vi "auto_alignment.vi"(0 "meter-visa":refnum<visa-resource-name>, 1 "xStart":dbl=264.0 format="%#_13g", 2 "yStart":dbl=123.0 format="%#_13g", 3 "NM-params":T1={"alpha"=1.0, "gamma"=2.0, "rho"=0.5, "sigma"=0.5, "simplex L"=0.5}, 5 "PD Values":cluster{"PD1":dbl, "PD2":dbl, "PD3":dbl}, 7 "stage-refs":T2, 9 "meter-error-in":errorcluster, 11 "stage-error-in":errorcluster) -> (4 "Optimized Location":dbl[](array[numeric]), 6 "Pts Tested":dbl[][](array[numeric]), 8 "std dev of simplex values":dbl, 10 "meter-error-out":errorcluster, 14 "run time (min)":dbl, 15 "stage-error-out":errorcluster)   [LabVIEW 2024]
uses:
  O:/DSG/Tyler/EIC/DIRC/daq/automated/Thorlabs.MotionControl.IntegratedStepperMotorsCLI.dll
  Thorlabs.MotionControl.IntegratedStepperMotorsCLI.dll
  O:/DSG/Tyler/EIC/DIRC/daq/automated/Thorlabs.MotionControl.Benchtop.StepperMotorCLI.dll
  Thorlabs.MotionControl.Benchtop.StepperMotorCLI.dll
  5b59031f-b1ff-41af-80a7-e72a33ebffa1.vi
  <vilib>/Array/Sort 2D Array - Pop Stack.vi
  <vilib>/Array/Sort 2D Array - Push Stack.vi
  5b59031f-b1ff-41af-80a7-e72a33ebffa1.vi/269d4b3b-47f5-49e3-8884-44851e4dd9d5.vi
  5b59031f-b1ff-41af-80a7-e72a33ebffa1.vi/6d99389c-673d-4efb-bf33-19b32bcf4cf8.vi
  <vilib>/Analysis/NI_AALBase.lvlib
panel:
  in  "nSamples":dbl=10.0 caption="# Samples"
  in  "simplex-limit":dbl=1e-06 caption="Simplex Length Convergence Goal" format="%#_13g"
  in  "value-limit":dbl=1e-08 caption="Value Convergence Goal" format="%#_13g"
  out "x_c":dbl[](array[numeric])
  out "x_e":dbl[](array[numeric])
  out "x_r":dbl[](array[numeric])
  out "x_o":dbl[](array[numeric])
  out "iterations timeout":bool
  out "simplex converge":bool
  out "value converge":bool
  out "simplex leg lengths":dbl[](array[numeric])
  in  "stop":bool
  # "centroid"
  # "reflection point"
  # "expansion point"
  # "contraction point"
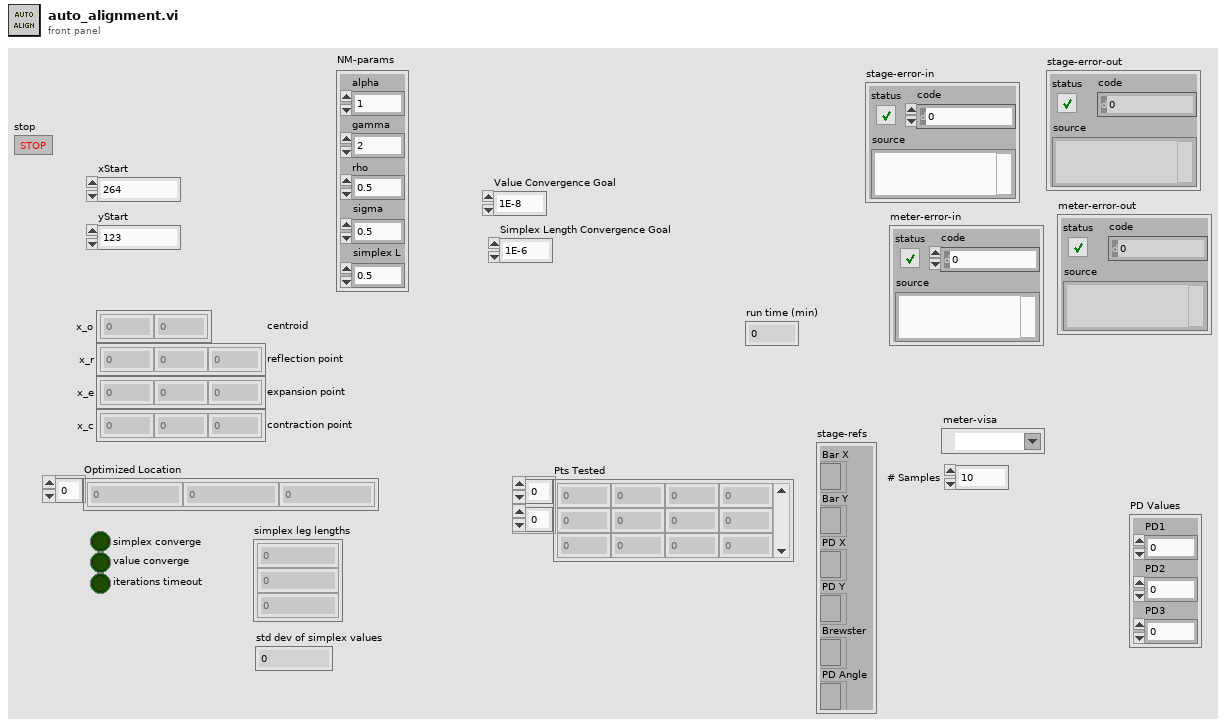
[diagram p1: front panel]
types:
  T1 = cluster{"alpha":dbl, "gamma":dbl, "rho":dbl, "sigma":dbl, "simplex L":dbl}
  T2 = cluster{"Bar X":refnum<k24>, "Bar Y":refnum<k24>, "PD X":refnum<k24>, "PD Y":refnum<k24>, "Brewster":refnum<k24>, "PD Angle":refnum<k24>}
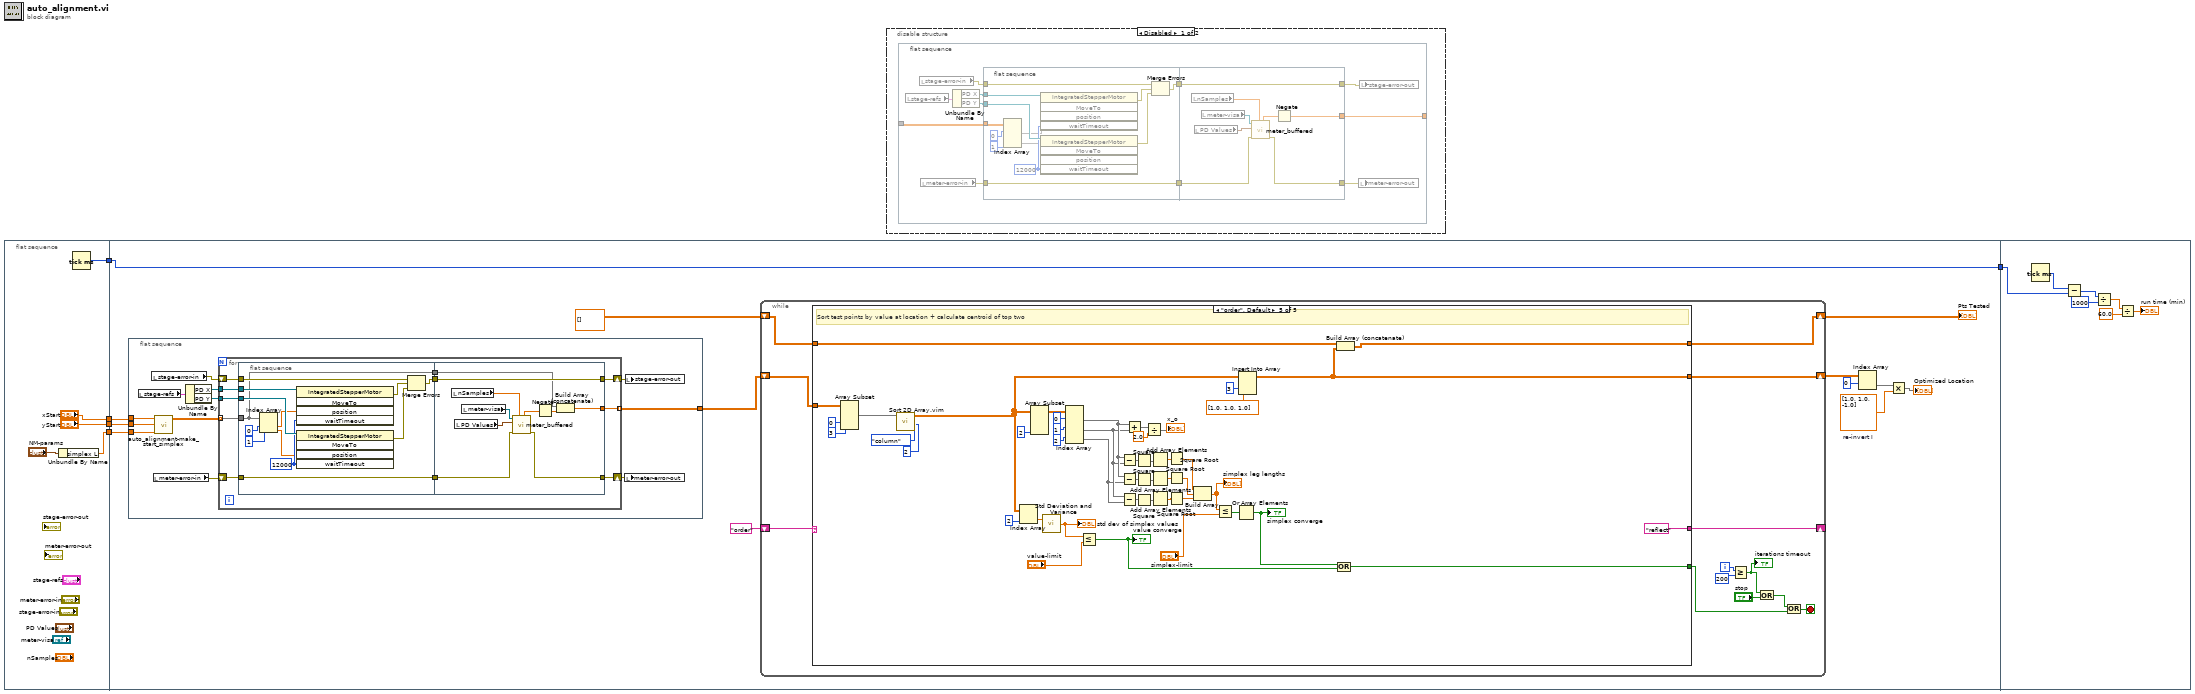
[diagram p0: block diagram]
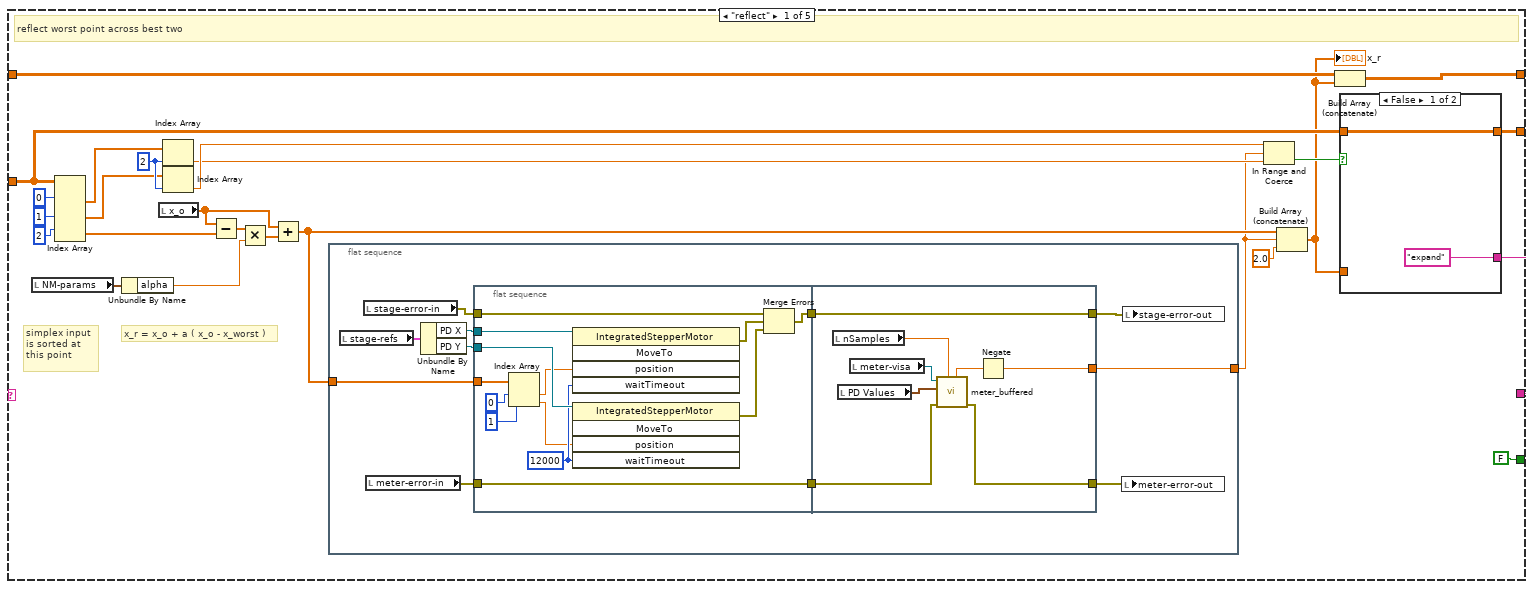
[diagram p3: hidden frame]
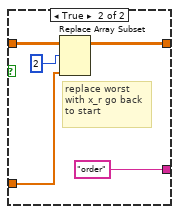
[diagram p4: hidden frame]
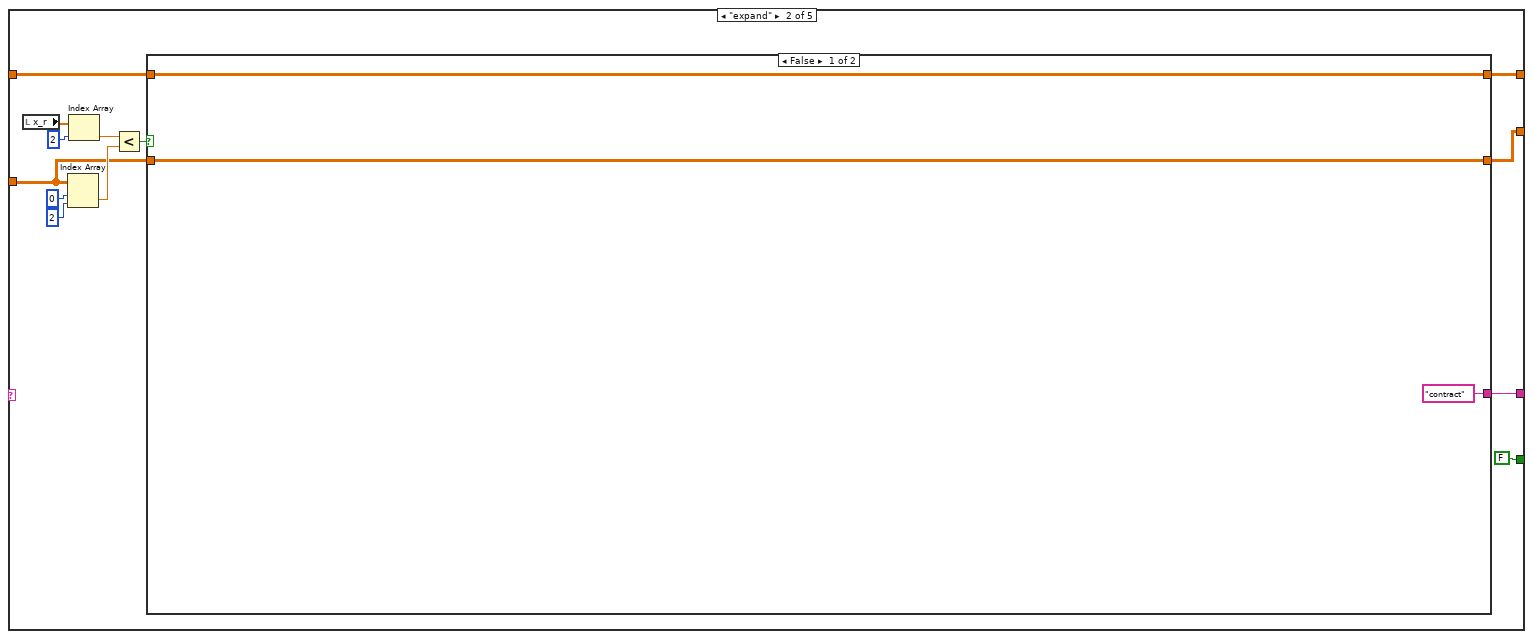
[diagram p5: hidden frame]
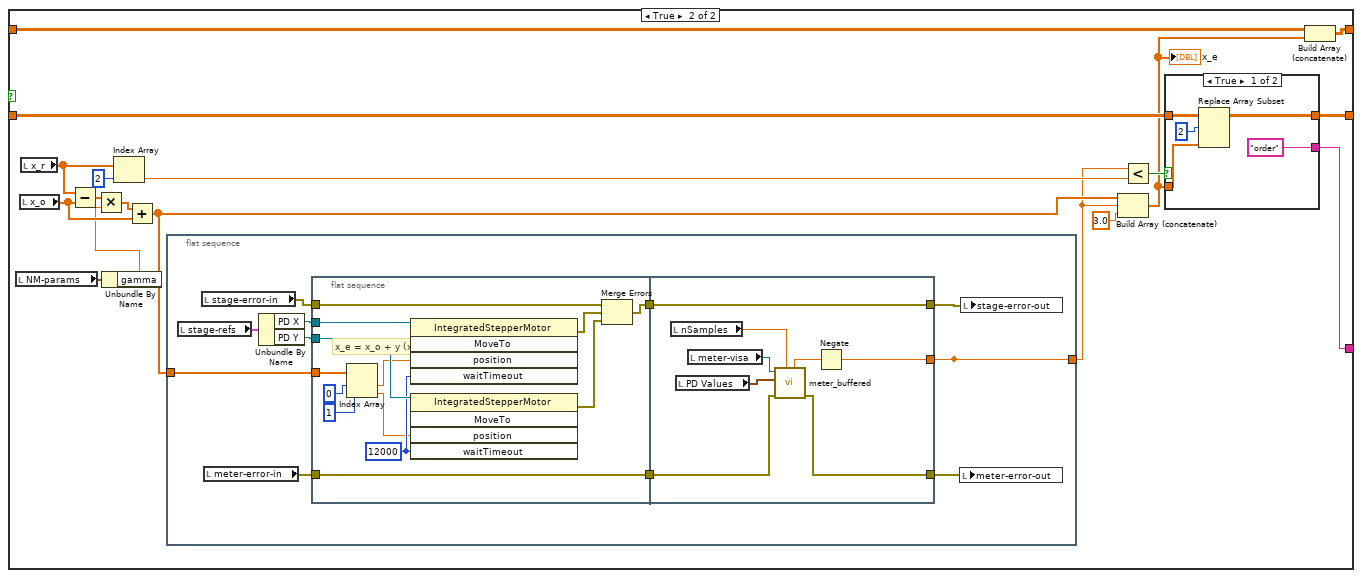
[diagram p6: hidden frame]
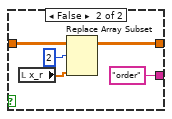
[diagram p7: hidden frame]
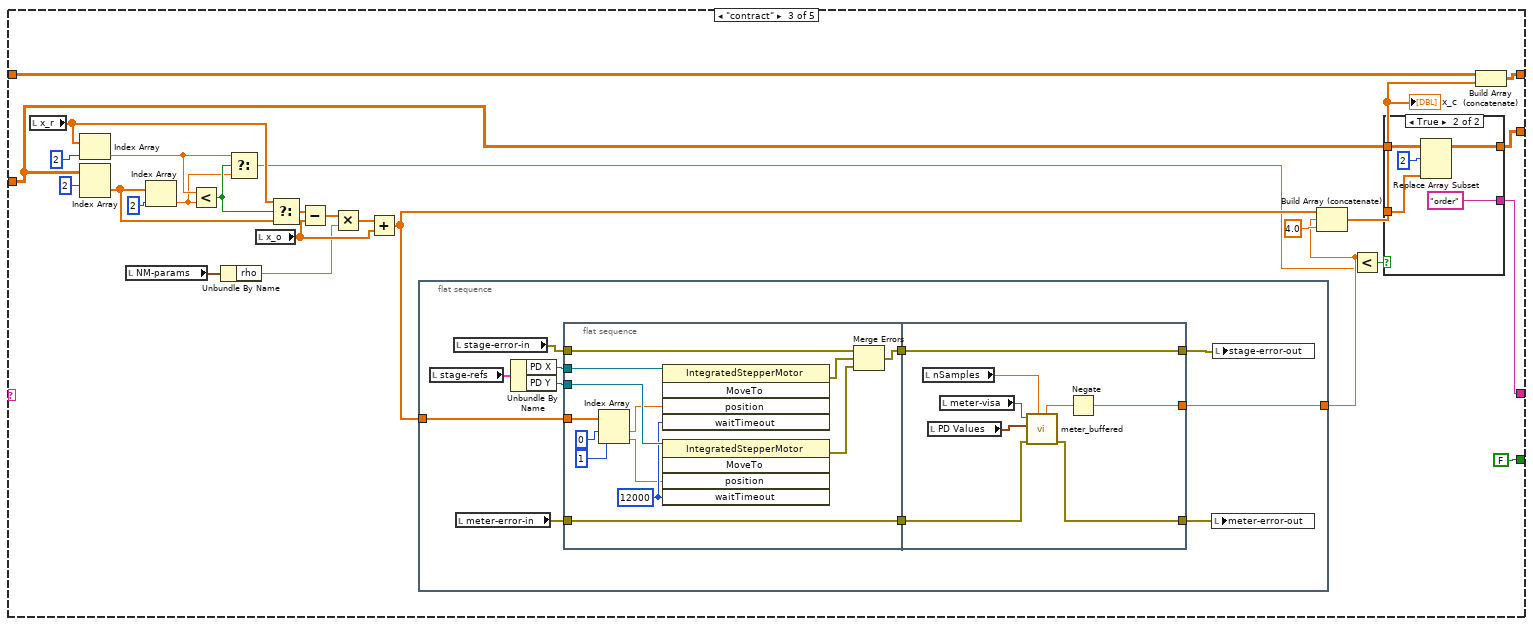
[diagram p8: hidden frame]
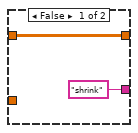
[diagram p9: hidden frame]
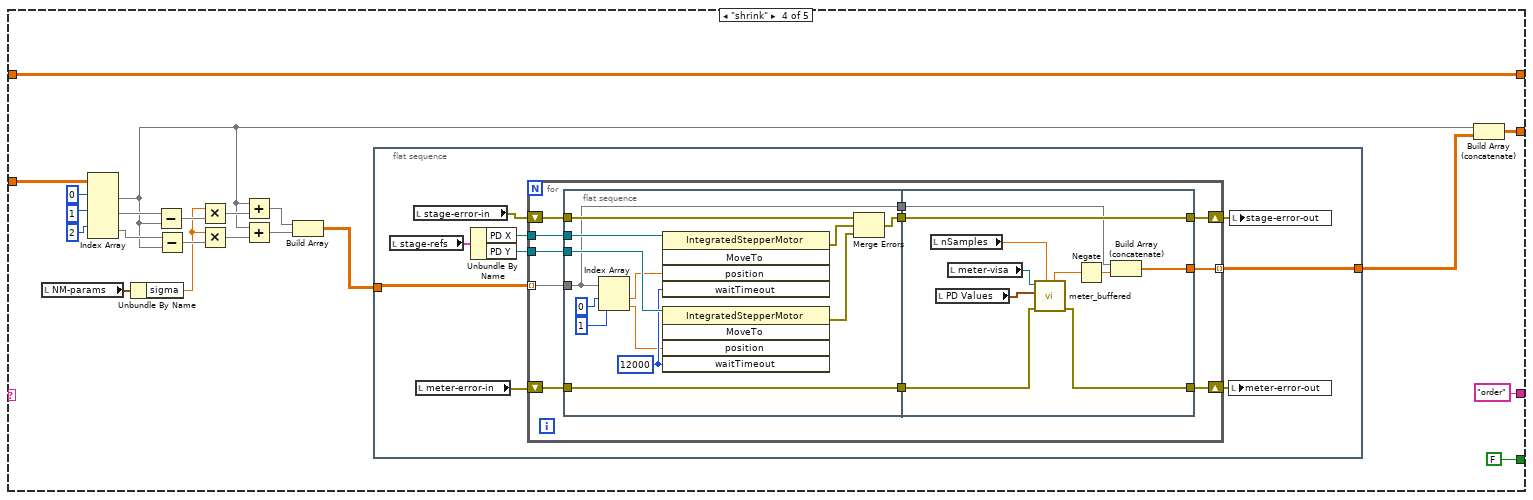
[diagram p10: hidden frame]
diagram:
  n1 = flat-sequence {
    tunnel: [w10] -> w5
    tunnel: ["yStart"] -> w3
    tunnel: ["xStart"] -> w2
    tunnel: [w6] -> w1
    tunnel: w5 -> [w21]
    tunnel: [w21] -> w4
    tunnel: w3 -> [w13]
    tunnel: w2 -> [w14]
    tunnel: w1 -> [w12]
    tunnel: w4 -> [w403]
    frame #0 {
      n2 = Unbundle By Name("NM-params") -> ("simplex L"=w6:dbl)
      n3 = Tick Count (ms)() -> (millisecond timer value=w10:u32)
    }
    frame #1 {
      w16 = dbl[] [1.0, 1.0, -1.0]  # re-invert I
      n4 = flat-sequence {
        tunnel: [w32] -> w15
        tunnel: w13 -> [w31]
        tunnel: w14 -> [w30]
        tunnel: w12 -> [w24]
        frame #0 {
          n5 = local read "stage-refs"() -> (w26:T2)
          n6 = local read "stage-error-in"() -> (w27:errorcluster)
          n7 = local read "meter-error-in"() -> (w25:errorcluster)
          n8 = call "auto_alignment-make_start_simplex.vi"("L"=w24, "yStart"=w31, "xStart"=w30) -> ("Array"=w33:dbl[][])  [unwired: 8 in]
          n9 = Unbundle By Name(w26) -> ("PD X"=w35:refnum<k24>, "PD Y"=w34:refnum<k24>)
          n10 = for {
            tunnel: w35 -> [w46]
            tunnel: w34 -> [w45]
            tunnel: w33 -> [w42] mode=indexing
            shift-right: [w40] -> w28
            shift-left: w27 -> [w44]
            tunnel: [w43] -> w32 mode=indexing
            shift-right: [w41] -> w29
            shift-left: w25 -> [w39]
            n11 = flat-sequence {
              tunnel: w46 -> [w57]
              tunnel: w45 -> [w56]
              tunnel: w44 -> [w50]
              tunnel: w42 -> [w48]
              tunnel: w39 -> [w47]
              tunnel: [w49] -> w38
              tunnel: [w48] -> w37
              tunnel: [w47] -> w36
              tunnel: [w69] -> w40
              tunnel: [w63] -> w41
              tunnel: [w66] -> w43
              tunnel: w38 -> [w69]
              tunnel: w37 -> [w65]
              tunnel: w36 -> [w64]
              frame #0 {
                w55 = 12000 ("waitTimeout")
                n12 = Index Array(array=w48, index #1=0 ("index"), index #2=1 ("index")) -> (element #1=w52:dbl, element #2=w51:dbl)
                n13 = invoke class="IntegratedStepperMotor" method="MoveTo"(reference=w57, "position"=w52, "waitTimeout"=w55) -> (error out=w59:errorcluster)  [unwired: 2 in, 4 out]
                n14 = invoke class="IntegratedStepperMotor" method="MoveTo"(reference=w56, "position"=w51, "waitTimeout"=w55) -> (error out=w58:errorcluster)  [unwired: 2 in, 4 out]
                n15 = Merge Errors(w50, w59, w58) -> (w49:errorcluster)
              }
              frame #1 {
                n16 = local read "nSamples"() -> (w62:dbl)
                n17 = local read "PD Values"() -> (w60:cluster{"PD1":dbl, "PD2":dbl, "PD3":dbl})
                n18 = local read "meter-visa"() -> (w61:refnum<visa-resource-name>)
                n19 = call "meter_buffered.vi"("Samples"=w62, "error in"=w64, "PD ranges"=w60, "meter-VISA"=w61) -> ("error out"=w63:errorcluster, "iCorr"=w67:dbl)  [unwired: 3 in, 3 out]
                n20 = Negate(x=w67) -> (-x=w68:dbl)
                n21 = Build Array (concatenate)(w65, w68) -> (w66:dbl[])
              }
            }
          }
          n22 = local write "meter-error-out"(w29) -> ()
          n23 = local write "stage-error-out"(w28) -> ()
        }
      }
      n24 = while {
        shift-right: [w80] -> w20
        shift-left: w15 -> [w79]
        shift-right: [w81] -> _
        shift-left: "order" -> [w82]
        shift-right: [w77] -> w11
        shift-left: dbl[][] [] -> [w78]
        i -> [w73]
        stop <- w71 stop-if-true
        n25 = case shown="\"order\", Default" w82 {
          tunnel: w79 -> [w93 w152 w235 w307 w389]
          tunnel: [FALSE FALSE FALSE FALSE w366] -> w75
          tunnel: [w92 w151 w236 w296 w355] -> w80
          tunnel: [w94 w150 w237 "order" "reflect"] -> w81
          tunnel: w78 -> [w90 w148 w231 w294 w354]
          tunnel: [w89 w147 w230 w294 w360] -> w77
          frame "reflect" {
            w101 = 2 ("index")
            # "simplex input\nis sorted at\nthis point"
            # "x_r = x_o + a ( x_o - x_worst )"
            # "reflect worst point across best two"
            n26 = local read "NM-params"() -> (w84:T1)
            n27 = Index Array(array=w93, index (row) #1=0 ("index (row)"), index (row) #2=1 ("index (row)"), index (row) #3=2 ("index (row)")) -> (element #1=w100:dbl[], element #2=w99:dbl[], element #3=w102:dbl[])  [unwired: 3 in]
            n28 = Unbundle By Name(w84) -> ("alpha"=w83:dbl)
            n29 = local read "x_o"() -> (w95:dbl[])
            n30 = Index Array(array=w100, index=w101) -> (element=w97:dbl)
            n31 = Index Array(array=w99, index=w101) -> (element=w98:dbl)
            n32 = Subtract(x=w95, y=w102) -> (x-y=w106:dbl[])
            n33 = Multiply(x=w106, y=w83) -> (x*y=w105:dbl[])
            n34 = Add(x=w95, y=w105) -> (x+y=w86:dbl[])
            n35 = flat-sequence {
              tunnel: [w108] -> w85
              tunnel: w86 -> [w109]
              frame #0 {
                n36 = local read "stage-refs"() -> (w113:T2)
                n37 = local read "stage-error-in"() -> (w114:errorcluster)
                n38 = local read "meter-error-in"() -> (w112:errorcluster)
                n39 = Unbundle By Name(w113) -> ("PD X"=w118:refnum<k24>, "PD Y"=w117:refnum<k24>)
                n40 = flat-sequence {
                  tunnel: w118 -> [w129]
                  tunnel: w117 -> [w128]
                  tunnel: w114 -> [w122]
                  tunnel: w109 -> [w120]
                  tunnel: w112 -> [w119]
                  tunnel: [w121] -> w111
                  tunnel: [w119] -> w110
                  tunnel: [w139] -> w115
                  tunnel: [w136] -> w116
                  tunnel: [w132] -> w108
                  tunnel: w111 -> [w139]
                  tunnel: w110 -> [w137]
                  frame #0 {
                    w127 = 12000 ("waitTimeout")
                    n41 = Index Array(array=w120, index #1=0 ("index"), index #2=1 ("index")) -> (element #1=w124:dbl, element #2=w123:dbl)
                    n42 = invoke class="IntegratedStepperMotor" method="MoveTo"(reference=w129, "position"=w124, "waitTimeout"=w127) -> (error out=w131:errorcluster)  [unwired: 2 in, 4 out]
                    n43 = invoke class="IntegratedStepperMotor" method="MoveTo"(reference=w128, "position"=w123, "waitTimeout"=w127) -> (error out=w130:errorcluster)  [unwired: 2 in, 4 out]
                    n44 = Merge Errors(w122, w131, w130) -> (w121:errorcluster)
                  }
                  frame #1 {
                    n45 = local read "nSamples"() -> (w135:dbl)
                    n46 = local read "PD Values"() -> (w133:cluster{"PD1":dbl, "PD2":dbl, "PD3":dbl})
                    n47 = local read "meter-visa"() -> (w134:refnum<visa-resource-name>)
                    n48 = call "meter_buffered.vi"("Samples"=w135, "error in"=w137, "PD ranges"=w133, "meter-VISA"=w134) -> ("error out"=w136:errorcluster, "iCorr"=w138:dbl)  [unwired: 3 in, 3 out]
                    n49 = Negate(x=w138) -> (-x=w132:dbl)
                  }
                }
                n50 = local write "meter-error-out"(w116) -> ()
                n51 = local write "stage-error-out"(w115) -> ()
              }
            }
            n52 = In Range and Coerce(upper limit=w98, x=w85, lower limit=w97) -> (In Range?=w96:bool)  [unwired: 1 out]
            n53 = Build Array (concatenate)(w86, w85, 2.0) -> (w88:dbl[])
            "x_r" <- w88
            n54 = Build Array (concatenate)(w90, w88) -> (w89:dbl[][])
            n55 = case shown="False" w96 {
              tunnel: ["expand" "order"] -> w94
              tunnel: w93 -> [w140 w146]
              tunnel: [w140 w143] -> w92
              tunnel: w88 -> [_ w144]
              frame False {
              }
              frame True {
                # "replace worst \nwith x_r go back\nto start"
                n56 = Replace Array Subset(array=w146, new element=w144, index (row)=2) -> (w143:dbl[][])  [unwired: 1 in]
              }
            }
          }
          frame "expand" {
            n57 = local read "x_r"() -> (w157:dbl[])
            n58 = Index Array(array=w152, index (row)=0, index (col)=2 ("disabled index (col)")) -> (element=w155:dbl)
            n59 = Index Array(array=w157, index=2) -> (element=w154:dbl)
            n60 = Less?(x=w154, y=w155) -> (x < y?=w153:bool)
            n61 = case shown="False" w153 {
              tunnel: w152 -> [w162 w173]
              tunnel: [w162 w172] -> w151
              tunnel: ["contract" w171] -> w150
              tunnel: w148 -> [w160 w170]
              tunnel: [w160 w169] -> w147
              frame False {
              }
              frame True {
                # "x_e = x_o + y (x _r - x _o)"
                n62 = local read "NM-params"() -> (w164:T1)
                n63 = local read "x_o"() -> (w178:dbl[])
                n64 = local read "x_r"() -> (w177:dbl[])
                n65 = Subtract(x=w177, y=w178) -> (x-y=w180:dbl[])
                n66 = Unbundle By Name(w164) -> ("gamma"=w163:dbl)
                n67 = Multiply(x=w180, y=w163) -> (x*y=w179:dbl[])
                n68 = Index Array(array=w177, index=2) -> (element=w175:dbl)
                n69 = Add(x=w179, y=w178) -> (x+y=w166:dbl[])
                n70 = flat-sequence {
                  tunnel: [w181] -> _
                  tunnel: w166 -> [w182]
                  tunnel: [w181] -> w165
                  frame #0 {
                    n71 = local read "stage-refs"() -> (w186:T2)
                    n72 = local read "stage-error-in"() -> (w187:errorcluster)
                    n73 = local read "meter-error-in"() -> (w185:errorcluster)
                    n74 = Unbundle By Name(w186) -> ("PD X"=w191:refnum<k24>, "PD Y"=w190:refnum<k24>)
                    n75 = flat-sequence {
                      tunnel: w191 -> [w202]
                      tunnel: w190 -> [w201]
                      tunnel: w187 -> [w195]
                      tunnel: w182 -> [w193]
                      tunnel: w185 -> [w192]
                      tunnel: [w194] -> w184
                      tunnel: [w192] -> w183
                      tunnel: [w212] -> w188
                      tunnel: [w209] -> w189
                      tunnel: [w205] -> w181
                      tunnel: w184 -> [w212]
                      tunnel: w183 -> [w210]
                      frame #0 {
                        w200 = 12000 ("waitTimeout")
                        n76 = Index Array(array=w193, index #1=0 ("index"), index #2=1 ("index")) -> (element #1=w197:dbl, element #2=w196:dbl)
                        n77 = invoke class="IntegratedStepperMotor" method="MoveTo"(reference=w202, "position"=w197, "waitTimeout"=w200) -> (error out=w204:errorcluster)  [unwired: 2 in, 4 out]
                        n78 = invoke class="IntegratedStepperMotor" method="MoveTo"(reference=w201, "position"=w196, "waitTimeout"=w200) -> (error out=w203:errorcluster)  [unwired: 2 in, 4 out]
                        n79 = Merge Errors(w195, w204, w203) -> (w194:errorcluster)
                      }
                      frame #1 {
                        n80 = local read "nSamples"() -> (w208:dbl)
                        n81 = local read "PD Values"() -> (w206:cluster{"PD1":dbl, "PD2":dbl, "PD3":dbl})
                        n82 = local read "meter-visa"() -> (w207:refnum<visa-resource-name>)
                        n83 = call "meter_buffered.vi"("Samples"=w208, "error in"=w210, "PD ranges"=w206, "meter-VISA"=w207) -> ("error out"=w209:errorcluster, "iCorr"=w211:dbl)  [unwired: 3 in, 3 out]
                        n84 = Negate(x=w211) -> (-x=w205:dbl)
                      }
                    }
                    n85 = local write "meter-error-out"(w189) -> ()
                    n86 = local write "stage-error-out"(w188) -> ()
                  }
                }
                n87 = Build Array (concatenate)(w166, w165, 3.0) -> (w168:dbl[])
                "x_e" <- w168
                n88 = Less?(x=w165, y=w175) -> (x < y?=w174:bool)
                n89 = case shown="True" w174 {
                  tunnel: w173 -> [w216 w221]
                  tunnel: w168 -> [w215 _]
                  tunnel: [w214 w220] -> w172
                  tunnel: ["order" "order"] -> w171
                  frame True {
                    n90 = Replace Array Subset(array=w216, new element=w215, index (row)=2) -> (w214:dbl[][])  [unwired: 1 in]
                  }
                  frame False {
                    n91 = local read "x_r"() -> (w218:dbl[])
                    n92 = Replace Array Subset(array=w221, new element=w218, index (row)=2) -> (w220:dbl[][])  [unwired: 1 in]
                  }
                }
                n93 = Build Array (concatenate)(w170, w168) -> (w169:dbl[][])
              }
            }
          }
          frame "contract" {
            n94 = local read "x_r"() -> (w245:dbl[])
            n95 = Index Array(array=w245, index=2) -> (element=w240:dbl)
            n96 = Index Array(array=w235, index (row)=2) -> (element=w244:dbl[])  [unwired: 1 in]
            n97 = local read "NM-params"() -> (w225:T1)
            n98 = Index Array(array=w244, index=2) -> (element=w239:dbl)
            n99 = Less?(x=w240, y=w239) -> (x < y?=w241:bool)
            n100 = Unbundle By Name(w225) -> ("rho"=w224:dbl)
            n101 = Select(t=w240, s=w241, f=w239) -> (s? t:f=w223:dbl)
            n102 = local read "x_o"() -> (w233:dbl[])
            n103 = Select(t=w245, s=w241, f=w244) -> (s? t:f=w243:dbl[])
            n104 = Subtract(x=w243, y=w233) -> (x-y=w242:dbl[])
            n105 = Multiply(x=w242, y=w224) -> (x*y=w234:dbl[])
            n106 = Add(x=w234, y=w233) -> (x+y=w227:dbl[])
            n107 = flat-sequence {
              tunnel: [w257] -> w226
              tunnel: w227 -> [w249]
              frame #0 {
                n108 = local read "stage-refs"() -> (w253:T2)
                n109 = local read "stage-error-in"() -> (w254:errorcluster)
                n110 = local read "meter-error-in"() -> (w252:errorcluster)
                n111 = Unbundle By Name(w253) -> ("PD X"=w259:refnum<k24>, "PD Y"=w258:refnum<k24>)
                n112 = flat-sequence {
                  tunnel: w259 -> [w270]
                  tunnel: w258 -> [w269]
                  tunnel: w254 -> [w263]
                  tunnel: w249 -> [w261]
                  tunnel: w252 -> [w260]
                  tunnel: [w262] -> w251
                  tunnel: [w260] -> w250
                  tunnel: [w280] -> w255
                  tunnel: [w277] -> w256
                  tunnel: [w273] -> w257
                  tunnel: w251 -> [w280]
                  tunnel: w250 -> [w278]
                  frame #0 {
                    w268 = 12000 ("waitTimeout")
                    n113 = Index Array(array=w261, index #1=0 ("index"), index #2=1 ("index")) -> (element #1=w265:dbl, element #2=w264:dbl)
                    n114 = invoke class="IntegratedStepperMotor" method="MoveTo"(reference=w270, "position"=w265, "waitTimeout"=w268) -> (error out=w272:errorcluster)  [unwired: 2 in, 4 out]
                    n115 = invoke class="IntegratedStepperMotor" method="MoveTo"(reference=w269, "position"=w264, "waitTimeout"=w268) -> (error out=w271:errorcluster)  [unwired: 2 in, 4 out]
                    n116 = Merge Errors(w263, w272, w271) -> (w262:errorcluster)
                  }
                  frame #1 {
                    n117 = local read "nSamples"() -> (w276:dbl)
                    n118 = local read "PD Values"() -> (w274:cluster{"PD1":dbl, "PD2":dbl, "PD3":dbl})
                    n119 = local read "meter-visa"() -> (w275:refnum<visa-resource-name>)
                    n120 = call "meter_buffered.vi"("Samples"=w276, "error in"=w278, "PD ranges"=w274, "meter-VISA"=w275) -> ("error out"=w277:errorcluster, "iCorr"=w279:dbl)  [unwired: 3 in, 3 out]
                    n121 = Negate(x=w279) -> (-x=w273:dbl)
                  }
                }
                n122 = local write "meter-error-out"(w256) -> ()
                n123 = local write "stage-error-out"(w255) -> ()
              }
            }
            n124 = Build Array (concatenate)(w227, w226, 4.0 ("array")) -> (w229:dbl[])
            "x_c" <- w229
            n125 = Less?(x=w226, y=w223) -> (x < y?=w238:bool)
            n126 = case shown="True" w238 {
              tunnel: ["shrink" "order"] -> w237
              tunnel: [w281 w283] -> w236
              tunnel: w235 -> [w281 w285]
              tunnel: w229 -> [_ w284]
              frame False {
              }
              frame True {
                n127 = Replace Array Subset(array=w285, new element=w284, index (row)=2) -> (w283:dbl[][])  [unwired: 1 in]
              }
            }
            n128 = Build Array (concatenate)(w231, w229) -> (w230:dbl[][])
          }
          frame "shrink" {
            n129 = local read "NM-params"() -> (w289:T1)
            n130 = Index Array(array=w307, index (row) #1=0 ("index (row)"), index (row) #2=1 ("index (row)"), index (row) #3=2 ("index (row)")) -> (element #1=w297:dbl[], element #2=w303:dbl[], element #3=w302:dbl[])  [unwired: 3 in]
            n131 = Unbundle By Name(w289) -> ("sigma"=w288:dbl)
            n132 = Subtract(x=w303, y=w297) -> (x-y=w300:dbl[])
            n133 = Subtract(x=w302, y=w297) -> (x-y=w301:dbl[])
            n134 = Multiply(x=w288, y=w300) -> (x*y=w299:dbl[])
            n135 = Multiply(x=w288, y=w301) -> (x*y=w298:dbl[])
            n136 = Add(x=w297, y=w299) -> (x+y=w293:dbl[])
            n137 = Add(x=w297, y=w298) -> (x+y=w292:dbl[])
            n138 = Build Array(w293, w292) -> (w291:dbl[][])
            n139 = flat-sequence {
              tunnel: [w315] -> w290
              tunnel: w291 -> [w309]
              frame #0 {
                n140 = local read "stage-refs"() -> (w311:T2)
                n141 = local read "stage-error-in"() -> (w312:errorcluster)
                n142 = local read "meter-error-in"() -> (w310:errorcluster)
                n143 = Unbundle By Name(w311) -> ("PD X"=w317:refnum<k24>, "PD Y"=w316:refnum<k24>)
                n144 = for {
                  tunnel: w317 -> [w328]
                  tunnel: w316 -> [w327]
                  tunnel: w309 -> [w324] mode=indexing
                  shift-right: [w322] -> w313
                  shift-left: w312 -> [w326]
                  tunnel: [w325] -> w315 mode=indexing
                  shift-right: [w323] -> w314
                  shift-left: w310 -> [w321]
                  n145 = flat-sequence {
                    tunnel: w328 -> [w339]
                    tunnel: w327 -> [w338]
                    tunnel: w326 -> [w332]
                    tunnel: w324 -> [w330]
                    tunnel: w321 -> [w329]
                    tunnel: [w331] -> w320
                    tunnel: [w330] -> w319
                    tunnel: [w329] -> w318
                    tunnel: [w351] -> w322
                    tunnel: [w345] -> w323
                    tunnel: [w348] -> w325
                    tunnel: w320 -> [w351]
                    tunnel: w319 -> [w347]
                    tunnel: w318 -> [w346]
                    frame #0 {
                      w337 = 12000 ("waitTimeout")
                      n146 = Index Array(array=w330, index #1=0 ("index"), index #2=1 ("index")) -> (element #1=w334:dbl, element #2=w333:dbl)
                      n147 = invoke class="IntegratedStepperMotor" method="MoveTo"(reference=w339, "position"=w334, "waitTimeout"=w337) -> (error out=w341:errorcluster)  [unwired: 2 in, 4 out]
                      n148 = invoke class="IntegratedStepperMotor" method="MoveTo"(reference=w338, "position"=w333, "waitTimeout"=w337) -> (error out=w340:errorcluster)  [unwired: 2 in, 4 out]
                      n149 = Merge Errors(w332, w341, w340) -> (w331:errorcluster)
                    }
                    frame #1 {
                      n150 = local read "nSamples"() -> (w344:dbl)
                      n151 = local read "PD Values"() -> (w342:cluster{"PD1":dbl, "PD2":dbl, "PD3":dbl})
                      n152 = local read "meter-visa"() -> (w343:refnum<visa-resource-name>)
                      n153 = call "meter_buffered.vi"("Samples"=w344, "error in"=w346, "PD ranges"=w342, "meter-VISA"=w343) -> ("error out"=w345:errorcluster, "iCorr"=w349:dbl)  [unwired: 3 in, 3 out]
                      n154 = Negate(x=w349) -> (-x=w350:dbl)
                      n155 = Build Array (concatenate)(w347, w350) -> (w348:dbl[])
                    }
                  }
                }
                n156 = local write "meter-error-out"(w314) -> ()
                n157 = local write "stage-error-out"(w313) -> ()
              }
            }
            n158 = Build Array (concatenate)(w297, w290) -> (w296:dbl[][])
          }
          frame "order", Default {
            # "Sort test points by value at location + calculate centroid of top two"
            n159 = Array Subset(array=w389, index (col)=0 ("index"), length (col)=3 ("length")) -> (w353:dbl[][])  [unwired: 2 in]
            n160 = call "Sort 2D Array.vim"("index"=2, "dimension to index (column)"=enum16{"column", "row"}."column", "2D array"=w353) -> ("sorted 2D array"=w358:dbl[][])  [unwired: 7 in, 1 out]
            n161 = Index Array(array=w358, index (col)=2 ("index")) -> (element=w383:dbl[])  [unwired: 1 in]
            n162 = Array Subset(array=w358, length (col)=2 ("length")) -> (w382:dbl[][])  [unwired: 3 in]
            n163 = call <vilib>:"Std Deviation and Variance.vi"("X"=w383) -> ("standard deviation"=w359:dbl)  [unwired: 1 in, 2 out]
            "std dev of simplex values" <- w359
            n164 = Index Array(array=w382, index (row) #1=0 ("index (row)"), index (row) #2=1 ("index (row)"), index (row) #3=2 ("index (row)")) -> (element #1=w363:dbl[], element #2=w362:dbl[], element #3=w361:dbl[])  [unwired: 3 in]
            n165 = Less Or Equal?(x=w359, y="value-limit") -> (x <= y?=w365:bool)
            "value converge" <- w365
            n166 = Subtract(x=w363, y=w362) -> (x-y=w380:dbl[])
            n167 = Subtract(x=w363, y=w361) -> (x-y=w372:dbl[])
            n168 = Subtract(x=w362, y=w361) -> (x-y=w375:dbl[])
            n169 = Add(x=w363, y=w362) -> (x+y=w387:dbl[])
            n170 = Square(x=w380) -> (x^2=w379:dbl[])
            n171 = Square(x=w372) -> (x^2=w376:dbl[])
            n172 = Square(x=w375) -> (x^2=w374:dbl[])
            n173 = Divide(x=w387, y=2.0) -> (x/y=→"x_o":dbl[])
            n174 = Add Array Elements(numeric array=w379) -> (sum=w378:dbl)
            n175 = Add Array Elements(numeric array=w376) -> (sum=w377:dbl)
            n176 = Add Array Elements(numeric array=w374) -> (sum=w373:dbl)
            n177 = Square Root(x=w378) -> (sqrt(x)=w369:dbl)
            n178 = Square Root(x=w377) -> (sqrt(x)=w370:dbl)
            n179 = Square Root(x=w373) -> (sqrt(x)=w371:dbl)
            n180 = Build Array(w369, w370, w371) -> (w368:dbl[])
            "simplex leg lengths" <- w368
            n181 = Less Or Equal?(x=w368, y="simplex-limit") -> (x <= y?=w367:bool[])
            n182 = Or Array Elements(Boolean array=w367) -> (logical OR=w364:bool)
            "simplex converge" <- w364
            n183 = Insert Into Array(array=w358, index (col)=3 ("disabled index (col)"), new element=dbl[] [1.0, 1.0, 1.0] ("new element/subarray")) -> (w355:dbl[][])  [unwired: 1 in]
            n184 = Build Array (concatenate)(w354, w355) -> (w360:dbl[][])
            n185 = Compound Arithmetic op=OR(w364, w365) -> (w366:bool)
          }
        }
        n186 = Greater Or Equal?(x=w73, y=200) -> (x >= y?=w72:bool)
        "iterations timeout" <- w72
        n187 = Compound Arithmetic op=OR(w72, "stop") -> (w70:bool)
        n188 = Compound Arithmetic op=OR(w70, w75) -> (w71:bool)
      }
      "Pts Tested" <- w11
      n189 = Index Array(array=w20, index (row)=0) -> (element=w17:dbl[])  [unwired: 1 in]
      n190 = Multiply(x=w17, y=w16) -> (x*y=→"Optimized Location":dbl[])
    }
    frame #2 {
      n191 = Tick Count (ms)() -> (millisecond timer value=w404:u32)
      n192 = Subtract(x=w404, y=w403) -> (x-y=w402:u32)
      n193 = Divide(x=w402, y=u32 1000) -> (x/y=w400:dbl)
      n194 = Divide(x=w400, y=60.0) -> (x/y=→"run time (min)":dbl)
    }
  }
  n195 = disable-structure shown="Disabled" {
    frame Disabled {
      n196 = flat-sequence {
        tunnel: [w413] -> _
        tunnel: [w405] -> _
        frame #0 {
          n197 = local read "stage-refs"() -> (w409:T2)
          n198 = local read "stage-error-in"() -> (w410:errorcluster)
          n199 = local read "meter-error-in"() -> (w408:errorcluster)
          n200 = Unbundle By Name(w409) -> ("PD X"=w415:refnum<k24>, "PD Y"=w414:refnum<k24>)
          n201 = flat-sequence {
            tunnel: w415 -> [w426]
            tunnel: w414 -> [w425]
            tunnel: w410 -> [w419]
            tunnel: [w417] -> w405
            tunnel: w408 -> [w416]
            tunnel: [w418] -> w407
            tunnel: [w416] -> w406
            tunnel: [w436] -> w411
            tunnel: [w433] -> w412
            tunnel: [w429] -> w413
            tunnel: w407 -> [w436]
            tunnel: w406 -> [w434]
            frame #0 {
              w424 = 12000 ("waitTimeout")
              n202 = Index Array(array=w417, index (row) #1=0 ("index"), index (row) #2=1 ("index")) -> (element #1=w421, element #2=w420)  [unwired: 2 in]
              n203 = invoke class="IntegratedStepperMotor" method="MoveTo"(reference=w426, "position"=w421, "waitTimeout"=w424) -> (error out=w428:errorcluster)  [unwired: 2 in, 4 out]
              n204 = invoke class="IntegratedStepperMotor" method="MoveTo"(reference=w425, "position"=w420, "waitTimeout"=w424) -> (error out=w427:errorcluster)  [unwired: 2 in, 4 out]
              n205 = Merge Errors(w419, w428, w427) -> (w418:errorcluster)
            }
            frame #1 {
              n206 = local read "nSamples"() -> (w432:dbl)
              n207 = local read "PD Values"() -> (w430:cluster{"PD1":dbl, "PD2":dbl, "PD3":dbl})
              n208 = local read "meter-visa"() -> (w431:refnum<visa-resource-name>)
              n209 = call "meter_buffered.vi"("Samples"=w432, "error in"=w434, "PD ranges"=w430, "meter-VISA"=w431) -> ("error out"=w433:errorcluster, "iCorr"=w435:dbl)  [unwired: 3 in, 3 out]
              n210 = Negate(x=w435) -> (-x=w429:dbl)
            }
          }
          n211 = local write "meter-error-out"(w412) -> ()
          n212 = local write "stage-error-out"(w411) -> ()
        }
      }
    }
    frame Enabled {
    }
  }
